vi "Calculate INL.vi"(11 "DNL":dbl[](array[numeric])) -> (3 "INL":dbl[](array[numeric]))   [LabVIEW 2021]
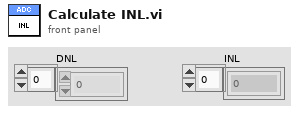
[diagram p1: front panel]
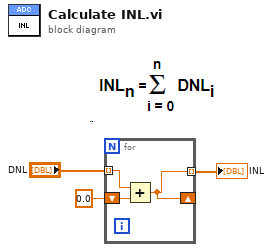
[diagram p0: block diagram]
diagram:
  n1 = for {
    tunnel: "DNL" -> [w5] mode=indexing
    shift-right: [w4] -> _
    shift-left: 0.0 -> [w6]
    tunnel: [w4] -> w3 mode=indexing
    n2 = Add(x=w5, y=w6) -> (x+y=w4:dbl)
  }
  "INL" <- w3
